vi "Initialize.vi"(8 "error in (no error)":errorcluster, 11 "Oscilloscope in":refnum<class "Oscilloscope.lvclass">) -> (0 "error out":errorcluster, 3 "Oscilloscope out":refnum<class "Oscilloscope.lvclass">)   [LabVIEW 2020, in "Oscilloscope.lvclass"]
doc: "VIRTUAL FUNCTION\n\nThis VI should be overwritten by methods using the specific initialization procedure for the respective child class."
uses:
  Oscilloscope.lvclass
  C:/Code Projects/CircuitExplorer/AnalogDiscoveryFunction/AnalogDiscoveryFunction.lvclass
  AnalogDiscoveryFunction/AnalogDiscoveryFunction.lvclass/AnalogDiscoveryFunction.ctl
  AnalogDiscoveryFunction/GetDeviceName.vi
  AnalogDiscoveryFunction/SetInstrumentHandle.vi
  Oscilloscope.lvclass/Oscilloscope.ctl
  <vilib>/DigilentWF/DigilentWF.lvlib
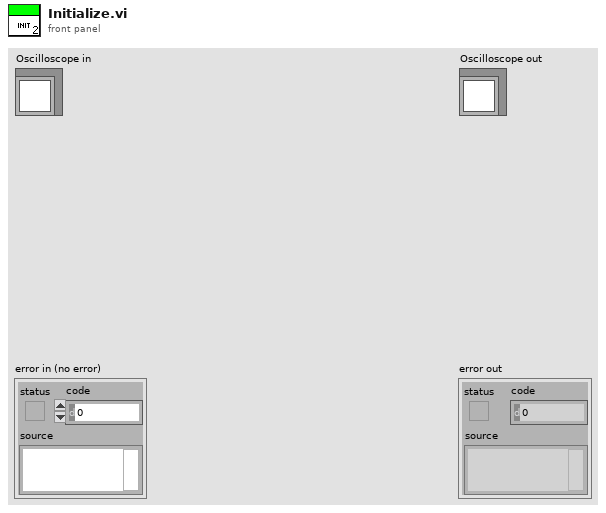
[diagram p1: front panel]
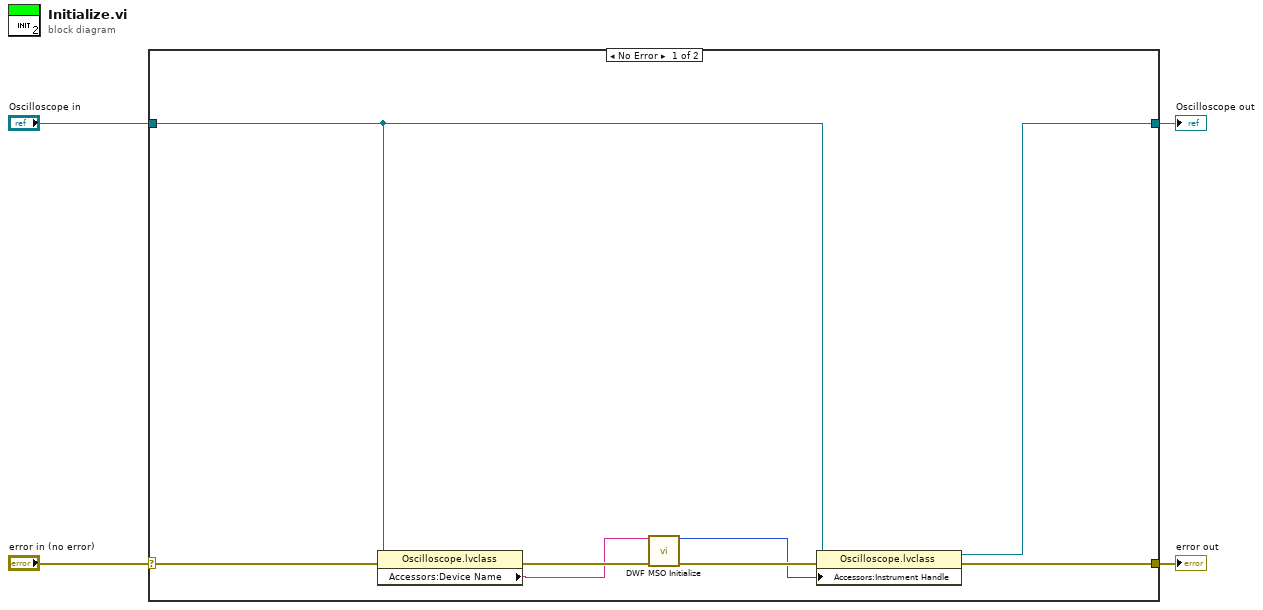
[diagram p0: block diagram]
diagram:
  n1 = case shown="No Error" "error in (no error)" {
    selector: "error in (no error)" -> [w12 w13]
    tunnel: [w8 w13] -> w3
    tunnel: [w6 w14] -> w1
    tunnel: "Oscilloscope in" -> [w7 w14]
    frame No Error {
      n2 = property class="Oscilloscope.lvclass"(reference=w7, error in=w12) -> (error out=w11:errorcluster, "Accessors:Device Name"=w10:string)  [unwired: 1 out]
      n3 = call <vilib>:"DWF MSO Initialize.vi"("Device Name"=w10, "Error In"=w11) -> ("Instrument Handle Out"=w5:u32, "Error Out"=w9:errorcluster)  [unwired: 12 in]
      n4 = property class="Oscilloscope.lvclass"(reference=w7, error in=w9, "Accessors:Instrument Handle"=w5) -> (reference out=w6:refnum<class "Oscilloscope.lvclass">, error out=w8:errorcluster)
    }
    frame Error {
    }
  }
  "error out" <- w3
  "Oscilloscope out" <- w1
